vi "CommandCycle.vi"(8 "Gripper Value R":dbl, 9 "Gripper Value L":dbl, 10 "Elevator Value":dbl, 11 "Teir Selection":T1) -> (3 "appended array":cluster{"States":T2, "Numeric":dbl}[](array[cluster]))   [LabVIEW 2017]
uses:
  Typedef/TeirNumber.ctl
  Elevator/Private/Typedef/Sequencer States.ctl
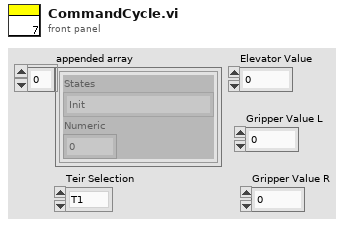
[diagram p1: front panel]
types:
  T1 = typedef "TeirNumber.ctl" = enum16{"T1", "T2", "T3", "T4", "T5", "T6"}
  T2 = typedef "Sequencer States.ctl" = enum16{"Init", "Set Elevator SP", "Set Gripper SP", "Wait For Elevator", "Wait For Gripper", ""}
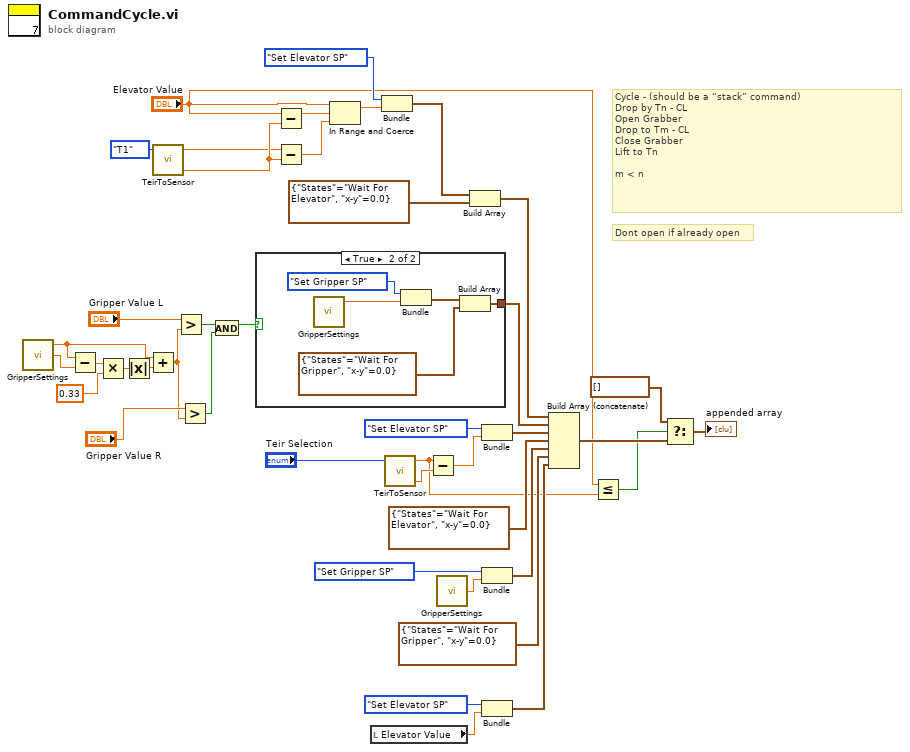
[diagram p0: block diagram]
diagram:
  # "Dont open if already open"
  # "Cycle - (should be a “stack” command)\nDrop by Tn - CL\nOpen Grabber\nDrop to Tm - CL\nClose Grabber\nLift to Tn\n\nm < n"
  n1 = call "GripperSettings.vi"() -> ("Open"=w28:dbl, "Close"=w23:dbl)  [unwired: 2 in, 1 out]
  n2 = Subtract(x=w28, y=w23) -> (x-y=w24:dbl)
  n3 = Multiply(x=w24, y=0.33) -> (x*y=w26:dbl)
  n4 = Absolute Value(x=w26) -> (abs(x)=w27:dbl)
  n5 = Add(x=w28, y=w27) -> (x+y=w9:dbl)
  n6 = call "TeirToSensor.vi"("Teir"=TeirNumber."T1" ("Enum")) -> ("CL"=w30:dbl, "Teir Height"=w29:dbl)  [unwired: 2 in, 1 out]
  n7 = Greater?(x="Gripper Value L", y=w9) -> (0:w14:bool)
  n8 = Greater?(x="Gripper Value R", y=w9) -> (0:w7:bool)
  n9 = And(x=w14, y=w7) -> (x .and. y?=w8:bool)
  n10 = case shown="True" w8 {
    tunnel: [_ w45] -> w15
    frame False {
    }
    frame True {
      n11 = call "GripperSettings.vi"() -> ("Open"=w46:dbl)  [unwired: 2 in, 2 out]
      n12 = Bundle("States"=Sequencer_States."Set Gripper SP", "Open"=w46) -> (w44:cluster{"States":T2, "Open":dbl})  [unwired: 1 in]
      n13 = Build Array(w44, cluster{"States":T2, "x-y":dbl} {"States"=enum."Wait For Gripper", "x-y"=0.0}) -> (w45:cluster{"States":T2, "x-y":dbl}[])
    }
  }
  n14 = Subtract(x="Elevator Value", y=w30) -> (x-y=w20:dbl)
  n15 = Subtract(x=w29, y=w30) -> (x-y=w19:dbl)
  n16 = In Range and Coerce(upper limit="Elevator Value", x=w20, lower limit=w19) -> (coerced(x)=w18:dbl)  [unwired: 1 out]
  n17 = local read "Elevator Value"() -> (w11:dbl)
  n18 = Bundle("States"=Sequencer_States."Set Elevator SP", "Elevator Value"=w18) -> (w17:cluster{"States":T2, "Elevator Value":dbl})  [unwired: 1 in]
  n19 = call "TeirToSensor.vi"("Teir"="Teir Selection") -> ("CL"=w40:dbl, "Teir Height"=w1:dbl)  [unwired: 2 in, 1 out]
  n20 = Subtract(x=w1, y=w40) -> (x-y=w39:dbl)
  n21 = call "GripperSettings.vi"() -> ("Close"=w34:dbl)  [unwired: 2 in, 2 out]
  n22 = Build Array(w17, cluster{"States":T2, "x-y":dbl} {"States"=enum."Wait For Elevator", "x-y"=0.0}) -> (w31:cluster{"States":T2, "x-y":dbl}[])
  n23 = Bundle("States"=Sequencer_States."Set Elevator SP", w39) -> (w37:cluster{"States":T2, dbl})  [unwired: 1 in]
  n24 = Bundle("States"=Sequencer_States."Set Gripper SP", "Close"=w34) -> (w35:cluster{"States":T2, "Close":dbl})  [unwired: 1 in]
  n25 = Bundle("States"=Sequencer_States."Set Elevator SP", "Elevator Value"=w11) -> (w42:cluster{"States":T2, "Elevator Value":dbl})  [unwired: 1 in]
  n26 = Build Array (concatenate)(w31, w15, w37, cluster{"States":T2, "x-y":dbl} {"States"=enum."Wait For Elevator", "x-y"=0.0}, w35, cluster{"States":T2, "x-y":dbl} {"States"=enum."Wait For Gripper", "x-y"=0.0}, w42) -> (w5:cluster{"States":T2, "Elevator Value":dbl}[])
  n27 = Less Or Equal?(x="Elevator Value", y=w1) -> (x <= y?=w4:bool)
  n28 = Select(t=cluster{"States":T2, "Elevator Value":dbl}[] [], s=w4, f=w5) -> (s? t:f=→"appended array":cluster{"States":T2, "Elevator Value":dbl}[])
